vi "Benchmark exprParser_eval.vi"(8 "error in (no error)":errorcluster, 10 "Iterations":i32, 11 "Expression":string) -> (0 "error out":errorcluster, 2 "x":dbl[](array[numeric]), 3 "y":dbl[](array[numeric]), 5 "dt average":dbl)   [LabVIEW 2015]
uses:
  <vilib>/gmath/NI_Gmath.lvlib
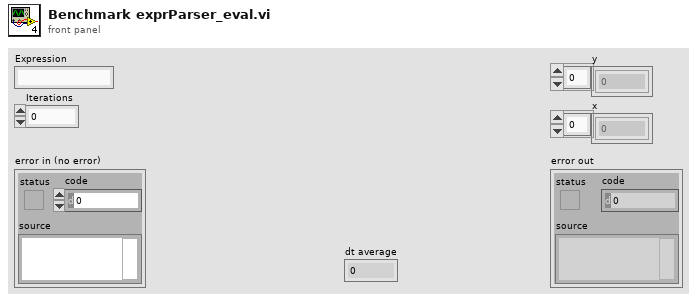
[diagram p1: front panel]
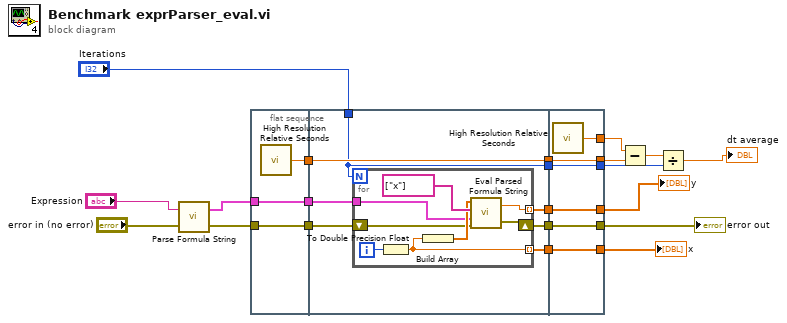
[diagram p0: block diagram]
diagram:
  n1 = call <vilib>:"Parse Formula String.vi"("error in (no error)"="error in (no error)", "formula"="Expression") -> ("error out"=w8:errorcluster, "Parsed Formula"=w6:cluster{"Table":i32[][], "Y Values":dbl[]})
  n2 = flat-sequence {
    tunnel: w8 -> [w23]
    tunnel: w6 -> [w24]
    tunnel: [w24] -> w19
    tunnel: [w23] -> w18
    tunnel: [w22] -> w13
    tunnel: w19 -> [w26]
    tunnel: w18 -> [w31]
    tunnel: [w30] -> w17
    tunnel: [w29] -> w16
    tunnel: [w28] -> w15
    tunnel: [w27] -> w14
    tunnel: w13 -> [w27]
    tunnel: "Iterations" -> [w25]
    tunnel: [w25] -> w3
    tunnel: [w43] -> w20
    tunnel: [w44] -> w21
    tunnel: [w45] -> w5
    tunnel: w17 -> [w45]
    tunnel: w16 -> [w44]
    tunnel: w15 -> [w43]
    tunnel: [w42] -> w11
    tunnel: w14 -> [w42]
    tunnel: [w41] -> w12
    tunnel: w3 -> [w40]
    tunnel: [w40] -> w2
    frame #0 {
      n3 = call <vilib>:"High Resolution Relative Seconds.vi"() -> ("relative seconds"=w22:dbl)
    }
    frame #1 {
      n4 = for {
        N: w25 -> [_]
        shift-right: [w32] -> w30
        shift-left: w31 -> [w35]
        tunnel: [w34] -> w29 mode=indexing
        tunnel: [w37] -> w28 mode=indexing
        tunnel: w26 -> [w33]
        i -> [w39]
        n5 = To Double Precision Float(number=w39) -> (double precision float=w37:dbl)
        n6 = Build Array(w37) -> (w36:dbl[])
        n7 = call <vilib>:"Eval Parsed Formula String.vi"("error in (no error)"=w35, "Parsed Formula"=w33, "Variables"=string[] ["x"], "X Values"=w36) -> ("error out"=w32:errorcluster, "y value"=w34:dbl)
      }
    }
    frame #2 {
      n8 = call <vilib>:"High Resolution Relative Seconds.vi"() -> ("relative seconds"=w41:dbl)
    }
  }
  n9 = Subtract(x=w12, y=w11) -> (x-y=w4:dbl)
  n10 = Divide(x=w4, y=w2) -> (x/y=→"dt average":dbl)
  "y" <- w21
  "x" <- w20
  "error out" <- w5
